vi "Nonce.vi"() -> (2 "delimiter":string)   [LabVIEW 2019]
uses:
  <vilib>/numeric/Random Number (Range) U64.vi
  <vilib>/numeric/sub_Random U32.vi
panel:
  out "string array":string[](array[string])
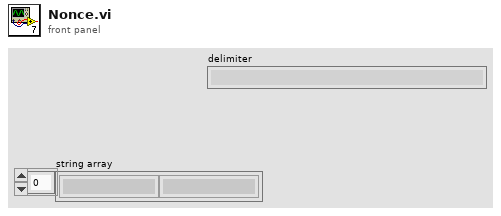
[diagram p1: front panel]
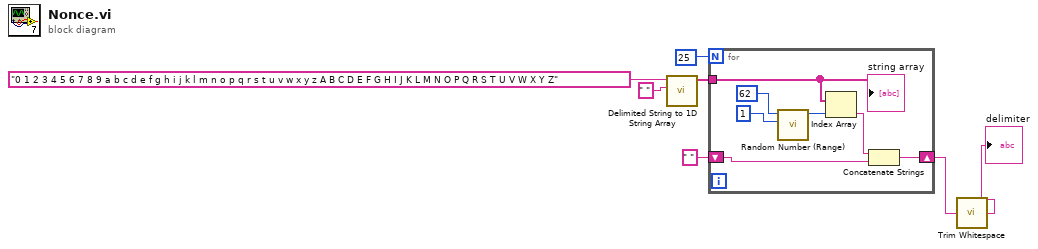
[diagram p0: block diagram]
diagram:
  n1 = call <vilib>:"Delimited String to 1D String Array.vi"("delimiter"=" ", "delimited string"="0 1 2 3 4 5 6 7 8 9 a b c d e f g h i j k l m n o p q r s t u v w x y z A B C D E F G H I J K L M N O P Q R S T U V W X Y Z") -> ("string array"=w4:string[])  [unwired: 9 in]
  n2 = for {
    N: 25 -> [_]
    tunnel: w4 -> [w12]
    shift-right: [w9] -> w2
    shift-left: " " ("delimiter") -> [w8]
    n3 = call-poly <vilib>:"Random Number (Range).vi"("lower bound (0)"=u64 1, "upper bound (100)"=u64 62) -> ("number"=w11:u64)  [unwired: 9 in]
    n4 = Index Array(array=w12, index=w11) -> (element=w10:string)
    n5 = Concatenate Strings(w10, w8) -> (w9:string)
    "string array" <- w12
  }
  n6 = call <vilib>:"Trim Whitespace.vi"("string"=w2) -> ("trimmed string"=→"delimiter":string)  [unwired: 1 in]
